vi "__AttrMap-GetValue2.vi"(8 "error in (no error)":errorcluster, 9 "Key":string, 11 "AttrMap in":T1) -> (0 "error out":errorcluster, 1 "found":bool, 2 "VAttributes":variant, 3 "AttrMap out":T1, 4 "OrignKey":string)   [LabVIEW 2019]
uses:
  Typedef/Def-AttrMap.ctl
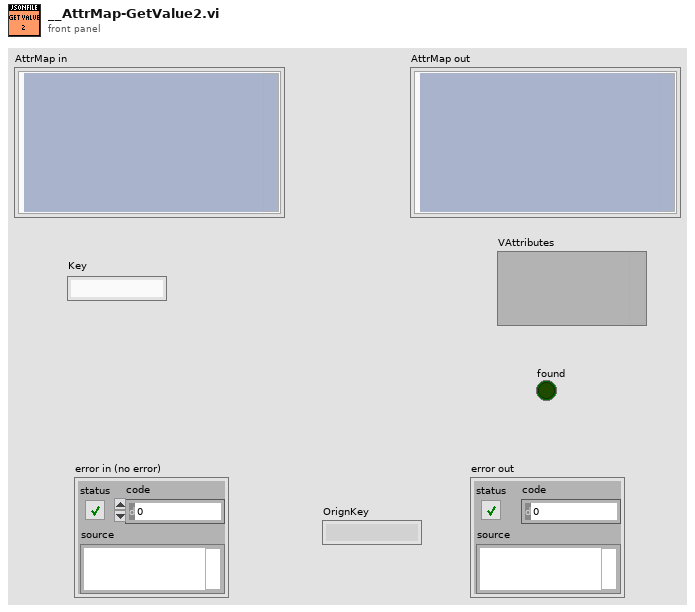
[diagram p1: front panel]
types:
  T1 = typedef "Def-AttrMap.ctl" = cluster{"Map":variant}
  T2 = typedef "Def-NameMap.ctl" = variant[]
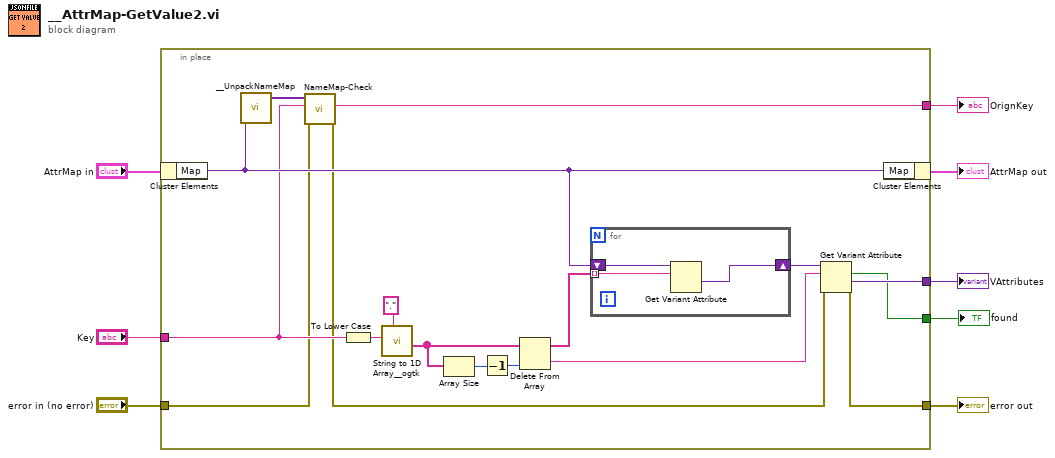
[diagram p0: block diagram]
diagram:
  n1 = in-place "In Place Element Structure" {
    in-place-border: [w11] -> w8
    in-place-border: "error in (no error)" -> [w14]
    in-place-border: "Key" -> [w15]
    in-place-border: [w12] -> w3
    in-place-border: [w10] -> w2
    in-place-border: [w9] -> w1
    n2 = in-place-cluster #1("AttrMap in") -> ("Map"=w17:variant)
    n3 = call "__UnpackNameMap.vi"("Map"=w17) -> ("NameMap"=w16:T2)  [unwired: 10 in]
    n4 = call "NameMap-Check.vi"("error in (no error)"=w14, "Name"=w15, "NameMap in"=w16) -> ("error out"=w13:errorcluster, "OriginName"=w10:string)  [unwired: 6 in, 1 out]
    n5 = To Lower Case(string=w15) -> (all lower case string=w23:string)
    n6 = call <userlib>:"String to 1D Array__ogtk.vi"("delimiter (Tab)"=".", "string"=w23) -> ("Array of Strings"=w20:string[])  [unwired: 9 in]
    n7 = Array Size(array=w20) -> (size(s)=w24:i32)
    n8 = Decrement(x=w24) -> (x-1=w18:i32)
    n9 = Delete From Array(array=w20, index=w18) -> (deleted portion=w21:string, array with subset deleted=w19:string[])  [unwired: 1 in]
    n10 = for {
      tunnel: w19 -> [w27] mode=indexing
      shift-right: [w26] -> w22
      shift-left: w17 -> [w28]
      n11 = Get Variant Attribute(Variant=w28, name=w27) -> (value=w26:variant)  [unwired: 2 in, 3 out]
    }
    n12 = Get Variant Attribute(Variant=w22, name=w21, error in=w13) -> (found=w9:bool, value=w12:variant, error out=w11:errorcluster)  [unwired: 1 in, 1 out]
    n13 = in-place-cluster #1("Map"=w17) -> (→"AttrMap out":T1)
  }
  "error out" <- w8
  "VAttributes" <- w3
  "OrignKey" <- w2
  "found" <- w1
